vi "updateGUIDisplayParams.vi"(8 "error in (no error)":errorcluster, 11 "Data Cluster in":T1) -> (0 "error out":errorcluster, 3 "Data Cluster out":T1)   [LabVIEW 2016]
uses:
  controls/UI Data.ctl
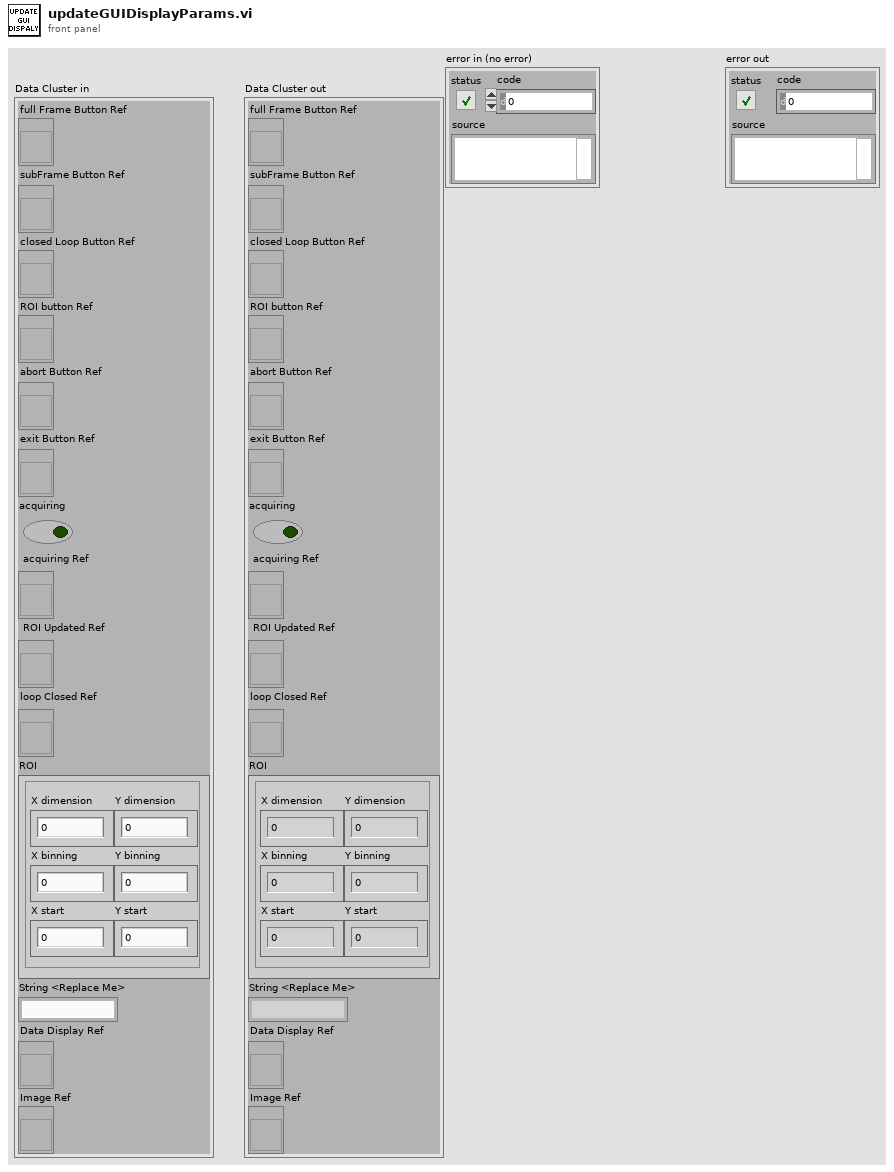
[diagram p1: front panel]
types:
  T1 = typedef "UI Data.ctl" = cluster{"full Frame Button Ref":refnum<vi>, "subFrame Button Ref":refnum<vi>, "closed Loop Button Ref":refnum<vi>, "ROI button Ref":refnum<vi>, "abort Button Ref":refnum<vi>, "exit Button Ref":refnum<vi>, "acquiring":bool, " acquiring Ref":refnum<vi>, " ROI Updated Ref":refnum<vi>, "loop Closed Ref":refnum<vi>, "ROI":cluster{"X dimension":i16, "Y dimension":i16, "X binning":i16, "Y binning":i16, "X start":i16, "Y start":i16}, "String <Replace Me>":string, "Data Display Ref":refnum<vi>, "Image Ref":refnum<vi>}
  T2 = enum8{"Enabled", "Disabled", "Disabled and Grayed Out"}
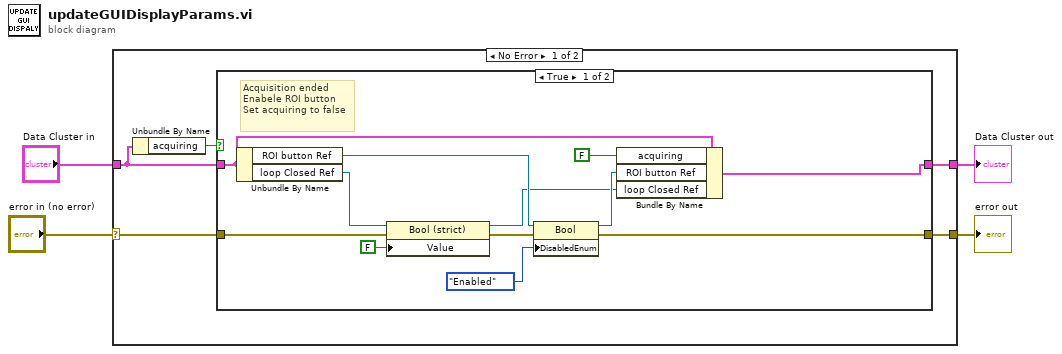
[diagram p0: block diagram]
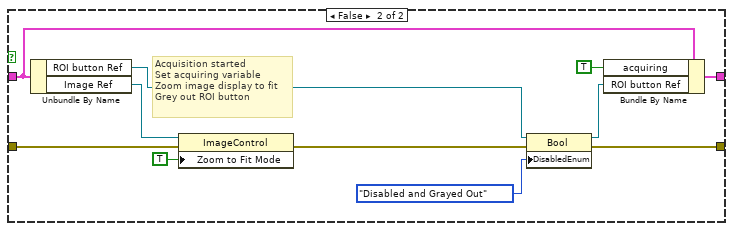
[diagram p2: hidden frame]
diagram:
  n1 = case shown="No Error" "error in (no error)" {
    selector: "error in (no error)" -> [w7 w33]
    tunnel: "Data Cluster in" -> [w9 w34]
    tunnel: [w6 w33] -> w2
    tunnel: [w5 w34] -> w1
    frame No Error {
      n2 = Unbundle By Name(w9) -> ("acquiring"=w8:bool)
      n3 = case shown="True" w8 {
        tunnel: w9 -> [w17 w27]
        tunnel: w7 -> [w13 w25]
        tunnel: [w15 w23] -> w6
        tunnel: [w16 w22] -> w5
        frame True {
          # "Acquisition ended\nEnabele ROI button\nSet acquiring to false"
          n4 = Unbundle By Name(w17) -> ("ROI button Ref"=w19:refnum<vi>, "loop Closed Ref"=w14:refnum<vi>)
          n5 = property class="Bool (strict)"(reference=w14, error in=w13, "Value"=FALSE) -> (reference out=w10:refnum<vi>, error out=w12:errorcluster)
          n6 = property class="Bool"(reference=w19, error in=w12, "DisabledEnum"=T2."Enabled" ("Disabled")) -> (reference out=w21:refnum<vi>, error out=w15:errorcluster)
          n7 = Bundle By Name(cluster=w17, "acquiring"=FALSE, "ROI button Ref"=w21, "loop Closed Ref"=w10) -> (w16:T1)
        }
        frame False {
          # "Acquisition started\nSet acquiring variable\nZoom image display to fit\nGrey out ROI button"
          n8 = Unbundle By Name(w27) -> ("ROI button Ref"=w30:refnum<vi>, "Image Ref"=w28:refnum<vi>)
          n9 = property class="ImageControl"(reference=w28, error in=w25, "Zoom to Fit Mode"=TRUE) -> (error out=w24:errorcluster)  [unwired: 1 out]
          n10 = property class="Bool"(reference=w30, error in=w24, "DisabledEnum"=T2."Disabled and Grayed Out" ("Disabled")) -> (reference out=w32:refnum<vi>, error out=w23:errorcluster)
          n11 = Bundle By Name(cluster=w27, "acquiring"=TRUE, "ROI button Ref"=w32) -> (w22:T1)
        }
      }
    }
    frame Error {
    }
  }
  "error out" <- w2
  "Data Cluster out" <- w1
